vi "获取最新数据.vi"(10 "时间标识":timestamp, 11 "组合框":string(combo)="氨氮") -> (2 "元素":T1, 3 "data":T2(array[cluster]))   [LabVIEW 2016, in "Alarm interface.lvlib" / "短信语音库.lvlib"]
uses:
  <vilib>/Utility/sysdir.llb/System Directory Type.ctl
  <vilib>/addons/database/Connection.llb/DB Tools Open Connec (String).vi
  <vilib>/addons/database/Connection.llb/Conn Execute.vi
  <vilib>/addons/database/Recordset.llb/Rec Fetch Recordset Data (R).vi
  <vilib>/addons/database/Recordset.llb/Rec Destroy - Connection.vi
  <vilib>/addons/database/_DB Variant To Data/Database Variant To Data.xnode
  <vilib>/addons/database/NI_Database_API.lvlib
panel:
  out "error out":errorcluster
  in  "error in (no error)":errorcluster
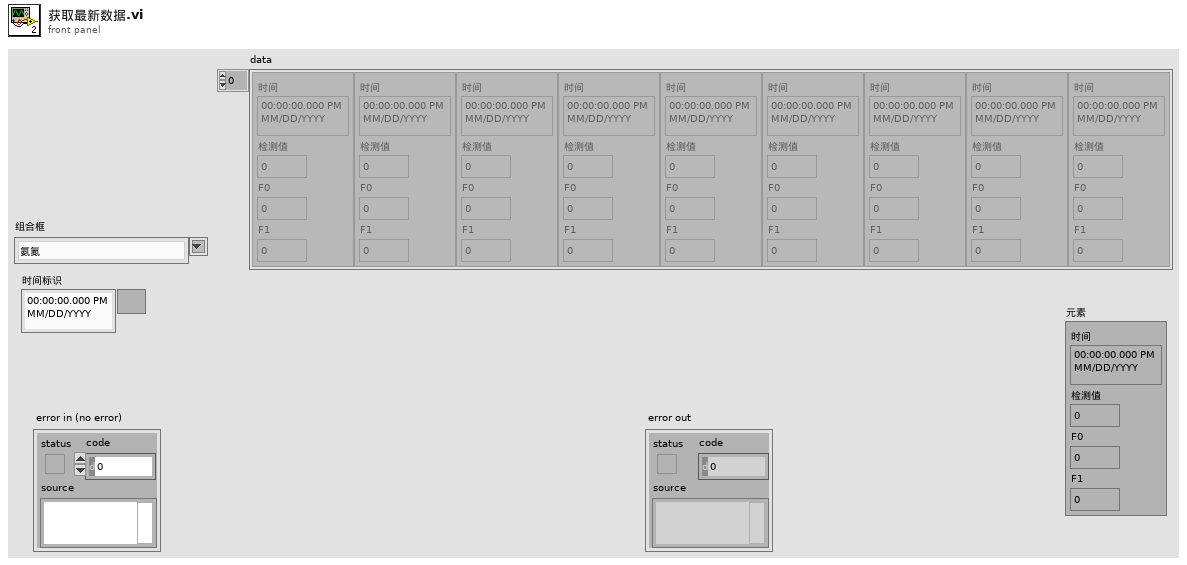
[diagram p1: front panel]
types:
  T1 = cluster{"时间":timestamp, "检测值":dbl, "F0":dbl, "F1":dbl}
  T2 = cluster{"时间":timestamp, "检测值":dbl, "F0":dbl, "F1":dbl}[]
  T3 = typedef "System Directory Type.ctl" = i32
  T4 = typedef "NI_Database_API.lvlib/Conn ObjectReference.ctl" = refnum<k1>
  T5 = typedef "NI_Database_API.lvlib/Rec ObjectReference.ctl" = refnum<k1>
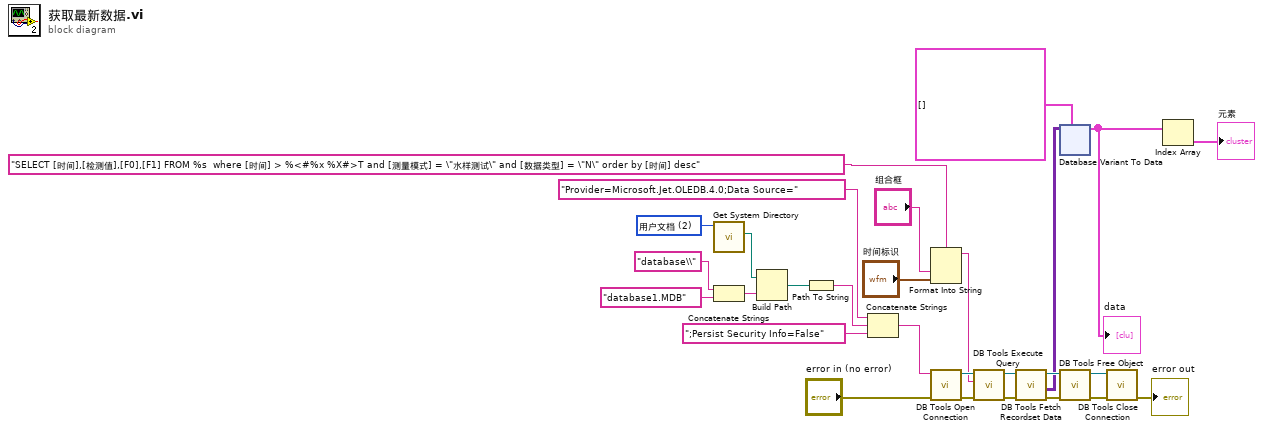
[diagram p0: block diagram]
diagram:
  w19 = T3 2 items=["用户目录"=0, "用户桌面"=1, "用户文档"=2, "用户应用程序数据"=3, "用户设置"=4, "用户临时目录"=5, "公共文档"=6, "公共应用程序数据"=7, "公共设置"=8, "公共缓存"=13, "系统核心库"=9, "系统安装库"=10, "应用程序文件"=11, "启动盘根目录"=12] ("system directory type")
  n1 = call <vilib>:"Get System Directory.vi"("system directory type"=w19) -> ("system directory"=w20:path)  [unwired: 10 in]
  n2 = Concatenate Strings("database\\" ("名称或相对路径"), "database1.MDB" ("database")) -> (w22:string)
  n3 = Build Path(base path=w20, name or relative path=w22) -> (appended path=w24:path)
  n4 = Path To String(path=w24) -> (string=w15:string)
  n5 = Concatenate Strings("Provider=Microsoft.Jet.OLEDB.4.0;Data Source=", w15, ";Persist Security Info=False") -> (w14:string)
  n6 = Format Into String(format string="SELECT [时间],[检测值],[F0],[F1] FROM %s  where [时间] > %<#%x %X#>T and [测量模式] = \"水样测试\" and [数据类型] = \"N\" order by [时间] desc" ("SQL query"), "组合框", "时间标识") -> (resulting string=w10:string)  [unwired: 2 in, 1 out]
  n7 = call-poly <vilib>:"DB Tools Open Connection.vi"("error in (no error)"="error in (no error)", "connection information"=w14) -> ("error out"=w25:errorcluster, "connection reference"=w18:T4)  [unwired: 6 in]
  n8 = call-poly <vilib>:"DB Tools Execute Query.vi"("error in (no error)"=w25, "SQL query"=w10, "connection reference"=w18) -> ("error out"=w13:errorcluster, "recordset reference"=w12:T5)  [unwired: 5 in]
  n9 = call-poly <vilib>:"DB Tools Fetch Recordset Data.vi"("error in (no error)"=w13, "recordset reference"=w12) -> ("error out"=w28:errorcluster, "recordset data"=w6:variant[][], "recordset reference out"=w27:T5)  [unwired: 3 in]
  n10 = xnode "Database Variant To Data"("database variant"=w6, "type"=T2 []) -> ("data"=w3:T2)  [unwired: 1 in, 1 out]
  "data" <- w3
  n11 = call-poly <vilib>:"DB Tools Free Object.vi"("error in (no error)"=w28, "recordset reference"=w27) -> ("error out"=w26:errorcluster, "connection reference"=w7:T4)  [unwired: 8 in]
  n12 = call <vilib>:"DB Tools Close Connection.vi"("error in (no error)"=w26, "connection reference"=w7) -> ("error out"=→"error out":errorcluster)  [unwired: 5 in]
  n13 = Index Array(array=w3) -> (element=→"元素":T1)  [unwired: 1 in]
